vi "string2boolean.vi"(1 "String":string) -> (0 "Boolean":bool)   [LabVIEW 2021]
doc: "This VI converts a string into a boolean.\nIs case insensitive and accepts the following string values:\ntrue, false, t, f, 1, 0, yes, no, y, n, on, off, enable, disable."
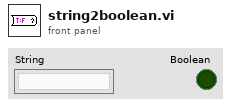
[diagram p1: front panel]
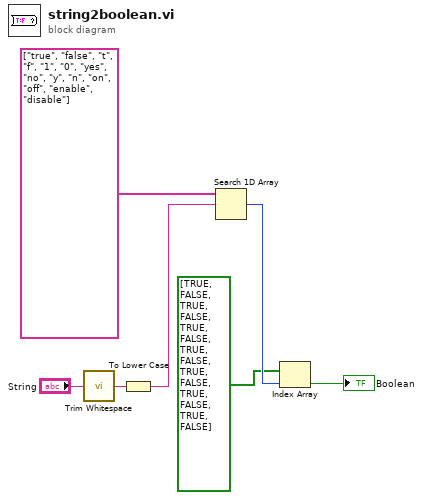
[diagram p0: block diagram]
diagram:
  n1 = call <vilib>:"Trim Whitespace.vi"("string"="String") -> ("trimmed string"=w1:string)  [unwired: 1 in]
  n2 = To Lower Case(string=w1) -> (all lower case string=w6:string)
  n3 = Search 1D Array(1D array=string[] ["true", "false", "t", "f", "1", "0", "yes", "no", "y", "n", "on", "off", "enable", "disable"], element=w6) -> (index of element=w4:i32)  [unwired: 1 out]
  n4 = Index Array(array=bool[] [TRUE, FALSE, TRUE, FALSE, TRUE, FALSE, TRUE, FALSE, TRUE, FALSE, TRUE, FALSE, TRUE, FALSE], index=w4) -> (element=→"Boolean":bool)
